vi "LVClass_ModalCoef GetData.vi"(0 "ModalCoef in":refnum<class "ModalCoef.lvclass">, 9 "Pupil.lvclass":refnum<class "Pupil.lvclass">, 11 "error in (no error)":errorcluster) -> (4 "ModalCoef out":refnum<class "ModalCoef.lvclass">, 6 "coef":sgl[](array[numeric]), 8 "index":u32[](array[numeric]), 10 "Pupil.lvclass (dup)":refnum<class "Pupil.lvclass">, 15 "error out":errorcluster)   [LabVIEW 2020, in "ModalCoef.lvclass"]
doc: "Get polynomial coefficients informations and values.\n\n--------------------------------------------------------------------------------\n\n<B>TypePhaseIn </B> : TypePhase phase mode reconstruction.\n<B>TypePhaseOut </B> : TypePhase phase mode reconstruction.\n<B>modalCoef </B> : ModalCoef object.\n<B>coef </B> : Array of modal coefficient values.\n<B>index </B> : Array of modal coefficient indices.\n<B>pupil </B> : pupil object.\n<B>ErrorIn </B> : Error\n<B>ErrorOut </B> : Error\n\n--------------------------------------------------------------------------------"
uses:
  ModalCoef.lvclass
  Pupil.lvclass
  ModalCoef.lvclass/ModalCoef.ctl
  LVClass_Pupil Read Pupil.vi
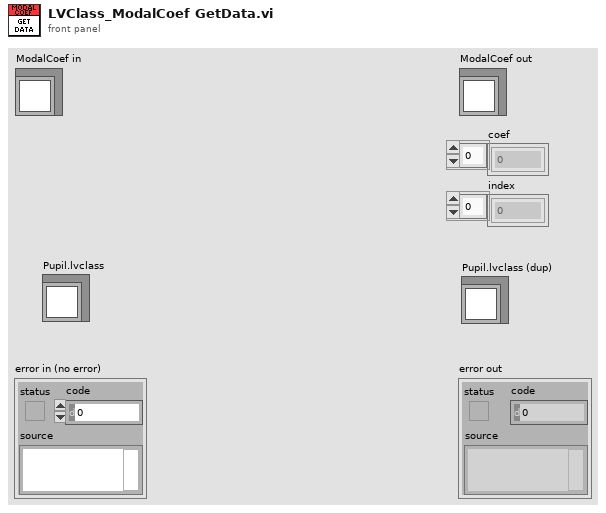
[diagram p1: front panel]
types:
  T1 = typedef "ClassID.ctl" = i64
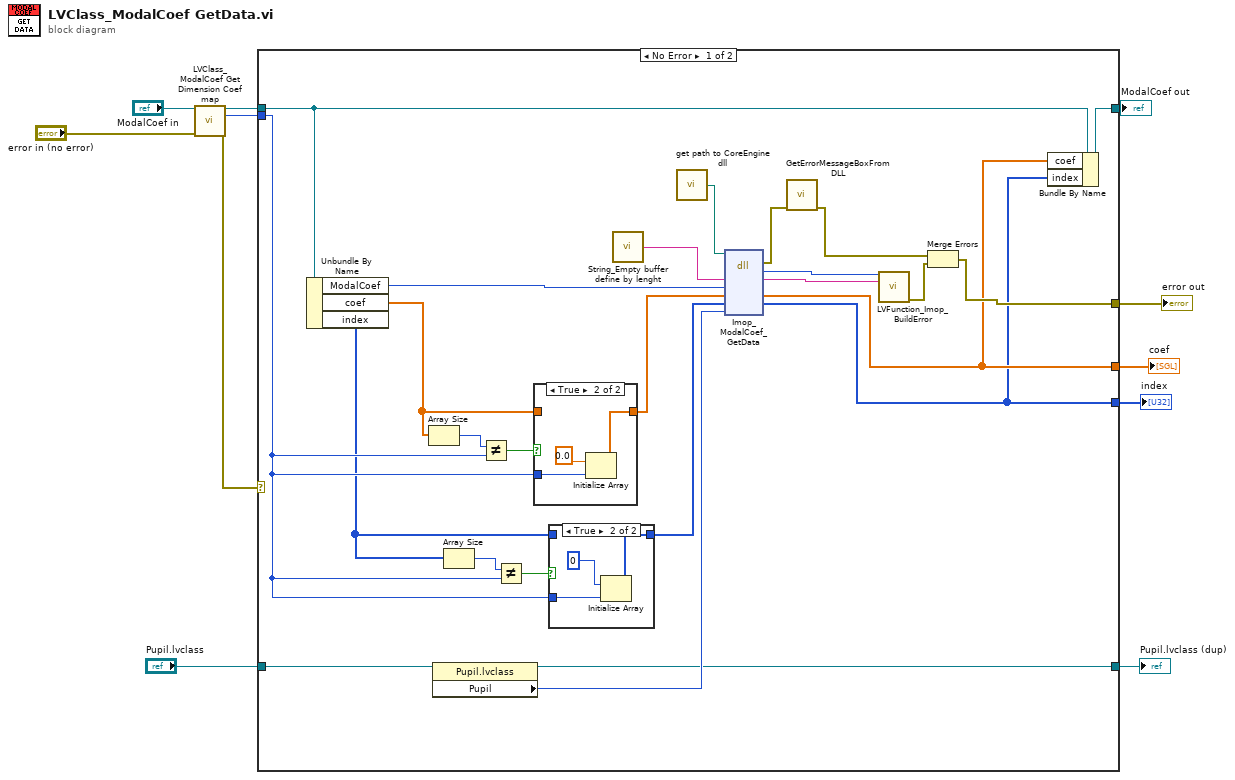
[diagram p0: block diagram]
diagram:
  n1 = call "LVClass_ModalCoef Get Dimension Coef map.vi"("ModalCoef in"="ModalCoef in", "error in (no error)"="error in (no error)") -> ("ModalCoef out"=w5:refnum<class "ModalCoef.lvclass">, "# of coef"=w2:i32, "error out"=w3:errorcluster)  [unwired: 11 in]
  n2 = case shown="No Error" w3 {
    selector: w3 -> [_ w47]
    tunnel: [w26 w47] -> w11
    tunnel: [w15 w46] -> w10
    tunnel: w5 -> [w16 w46]
    tunnel: "Pupil.lvclass" -> [w35 w45]
    tunnel: [w14 _] -> w8
    tunnel: [w13 _] -> w7
    tunnel: w2 -> [w19 _]
    tunnel: [w12 w45] -> w1
    frame No Error {
      n3 = Unbundle By Name(w16) -> ("ModalCoef"=w36:T1, "coef"=w25:sgl[], "index"=w18:u32[])
      n4 = Array Size(array=w25) -> (size(s)=w24:i32)
      n5 = property class="Pupil.lvclass"(reference=w35) -> (reference out=w12:refnum<class "Pupil.lvclass">, "Pupil"=w34:T1)  [unwired: 1 in, 1 out]
      n6 = Array Size(array=w18) -> (size(s)=w20:i32)
      n7 = Not Equal?(x=w24, y=w19) -> (x != y?=w23:bool)
      n8 = Not Equal?(x=w20, y=w19) -> (x != y?=w21:bool)
      n9 = case shown="True" w23 {
        tunnel: [w41 w43] -> w22
        tunnel: w19 -> [_ w44]
        tunnel: w25 -> [w41 _]
        frame False {
        }
        frame True {
          n10 = Initialize Array(sgl 0.0, w44) -> (w43:sgl[])
        }
      }
      n11 = case shown="True" w21 {
        tunnel: [w37 w39] -> w17
        tunnel: w19 -> [_ w40]
        tunnel: w18 -> [w37 _]
        frame False {
        }
        frame True {
          n12 = Initialize Array(u32 0, w40) -> (w39:u32[])
        }
      }
      n13 = call "String_Empty buffer define by lenght.vi"() -> ("Empty buffer"=w33:string)  [unwired: 1 in]
      n14 = call "get path to CoreEngine dll.vi"() -> ("path to wavekit library"=w30:path)  [unwired: 14 in, 1 out]
      n15 = dll-call lib="D:/2_trunk/Soft_haso/ImOpCoreEngine4_LV2011/DLLs/ImopEngine4_vc100.dll" fn="Imop_ModalCoef_GetData"(path in=w30, "message"=w33, "ModalCoef"=w36, "coef"=w22, "index"=w17, "pupil"=w34) -> (error out=w29:errorcluster, "return type"=w31:i32, "message"=w32:string, "coef"=w14:sgl[], "index"=w13:u32[])  [unwired: 4 in, 1 out]
      n16 = call "GetErrorMessageBoxFromDLL.vi"("error IN"=w29) -> ("error OUT"=w28:errorcluster)  [unwired: 10 in]
      n17 = call "LVFunction_Imop_BuildError.vi"("code"=w31, "String to Prepend to source (\"\")"=w32) -> ("error out"=w27:errorcluster)  [unwired: 13 in]
      n18 = Merge Errors(w28, w27) -> (w26:errorcluster)
      n19 = Bundle By Name(cluster=w16, "coef"=w14, "index"=w13) -> (w15:refnum<class "ModalCoef.lvclass">)
    }
    frame Error {
    }
  }
  "error out" <- w11
  "ModalCoef out" <- w10
  "index" <- w7
  "coef" <- w8
  "Pupil.lvclass (dup)" <- w1
